vi "WritePickeringConfig.vi"(8 "error in (no error)":errorcluster, 10 "Pickering Config":T1) -> (0 "Error Out":errorcluster)   [LabVIEW 2016, in "pickering.lvclass"]
uses:
  pickering.lvclass
  Typedefs/PickeringConfig-Cluster.ctl
  Typedefs/PickeringXConfig-Cluster.ctl
  Typedefs/PickeringYConfig-Cluster.ctl
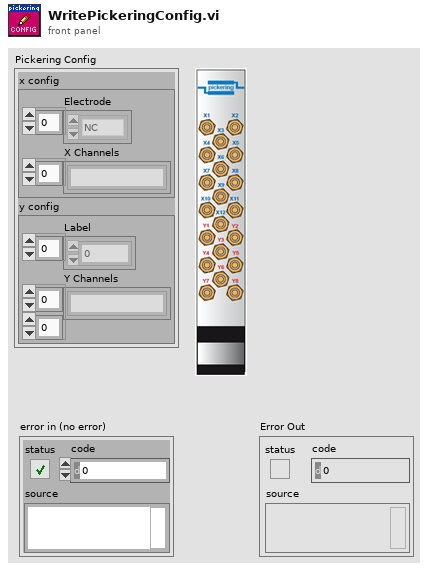
[diagram p1: front panel]
types:
  T1 = typedef "pickering.lvclass/PickeringConfig-Cluster.ctl" = cluster{"x config":T2, "y config":T3}
  T2 = typedef "pickering.lvclass/PickeringXConfig-Cluster.ctl" = cluster{"Electrode":enum16{"NC", "26", "27", "28", "1", "2", "3", "4", "5", "6", "7", "8", "9", "10", "11", "12", "13", "14", "15", "16", "17", "18", "19", "20", "21", "22", "23", "24", "25"}[], "X Channels":string[]}
  T3 = typedef "pickering.lvclass/PickeringYConfig-Cluster.ctl" = cluster{"Label":u16[], "Y Channels":string[][]}
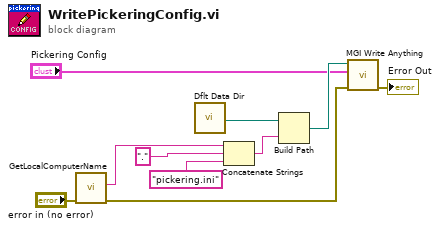
[diagram p0: block diagram]
diagram:
  n1 = call <userlib>:"GetLocalComputerName.vi"("error in (no error)"="error in (no error)") -> ("error out"=w6:errorcluster, "Name"=w5:string)  [unwired: 8 in, 1 out]
  n2 = call <vilib>:"Dflt Data Dir.vi"() -> ("App:Default Data Directory"=w10:path)
  n3 = Concatenate Strings(w5, "." ("string"), "pickering.ini" ("name or relative path")) -> (w7:string)
  n4 = Build Path(base path=w10, name or relative path=w7) -> (appended path=w9:path)
  n5 = call <userlib>:"MGI Write Anything.vi"("Error In"=w6, "Anything"="Pickering Config", "Path (dialog)"=w9) -> ("Error Out"=→"Error Out":errorcluster)  [unwired: 6 in, 2 out]
